vi "Set Properties During Initialization.vi"(6 "Constants VI":path, 8 "error in (no error)":errorcluster, 10 "Properties":T1[](array[typedef]), 11 "Path to VI":path) -> (0 "error out":errorcluster)   [LabVIEW 2017, in "NIVS_Consolidated_CDW_MetaDataObj.lvclass"]
uses:
  NIVS_Consolidated_CDW_MetaDataObj.lvclass
  Property Information.ctl
  <vilib>/Utility/traverseref.llb/TRef TravTarget.ctl
  <vilib>/Utility/traverseref.llb/VI Scripting - Traverse.lvlib
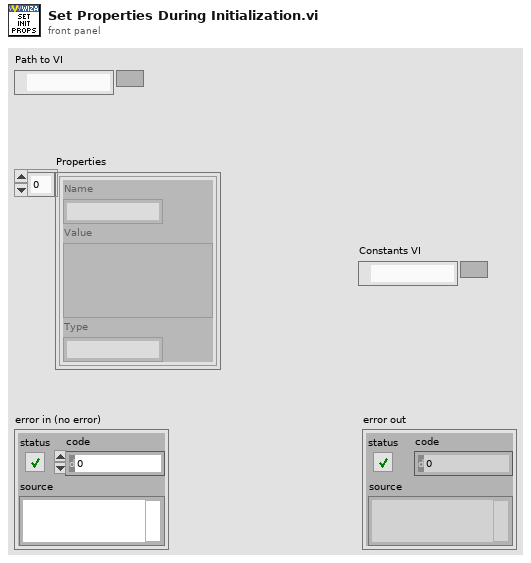
[diagram p1: front panel]
types:
  T1 = typedef "NIVS_Consolidated_CDW_MetaDataObj.lvclass/Property Information.ctl" = cluster{"Name":string, "Value":variant, "Type":string}
  T2 = typedef "TRef TravTarget.ctl" = enum16{"FP", "BD", "Other"}
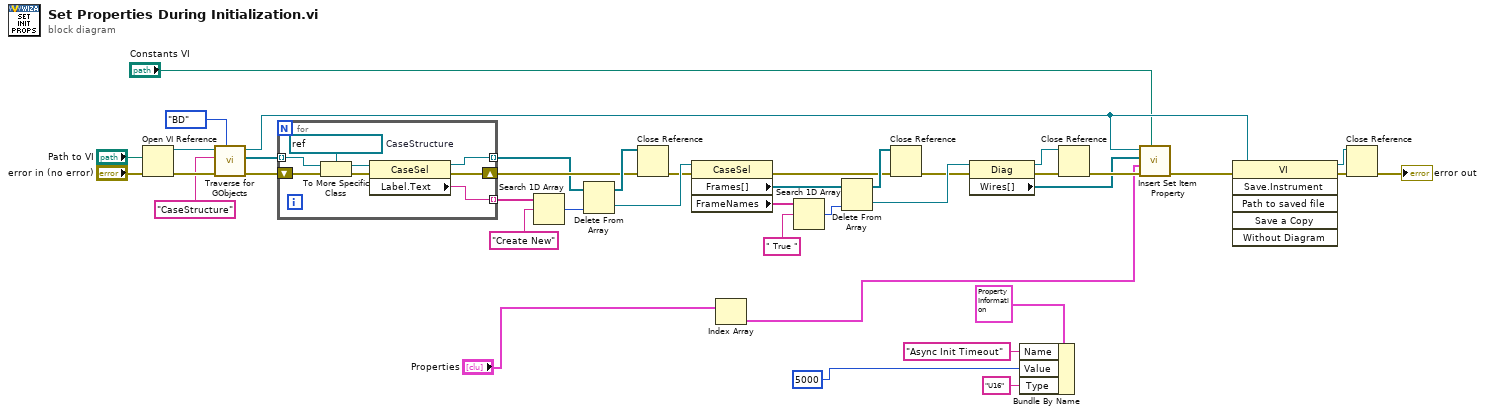
[diagram p0: block diagram]
diagram:
  n1 = Open VI Reference(vi path="Path to VI", error in (no error)="error in (no error)") -> (vi reference=w38:refnum<vi>, error out=w40:errorcluster)  [unwired: 4 in]
  n2 = call <vilib>:"Traverse for GObjects.vi"("Traverse Target"=TRef_TravTarget."BD", "error in (no error)"=w40, "Class Name"="CaseStructure", "VI Refnum"=w38) -> ("error out"=w36:errorcluster, "References"=w33:refnum<vi>[], "dup VI Refnum"=w6:refnum<vi>)  [unwired: 4 in, 1 out]
  n3 = for {
    tunnel: w33 -> [w46] mode=indexing
    shift-right: [w45] -> w30
    shift-left: w36 -> [w47]
    tunnel: [w42] -> w35 mode=indexing
    tunnel: [w41] -> w23 mode=indexing
    w48 = refnum<vi> refnum  # CaseStructure
    n4 = To More Specific Class(target class=w48, reference=w46, error in=w47) -> (specific class reference=w43:refnum<vi>, error out=w44:errorcluster)
    n5 = property class="CaseSel"(reference=w43, error in=w44) -> (reference out=w41:refnum<vi>, error out=w45:errorcluster, "Label.Text"=w42:string)
  }
  n6 = Search 1D Array(1D array=w35, element="Create New") -> (index of element=w31:i32)  [unwired: 1 in]
  n7 = Delete From Array(array=w23, index=w31) -> (deleted portion=w22:refnum<vi>, array with subset deleted=w32:refnum<vi>[])  [unwired: 1 in]
  n8 = Close Reference(reference=w32, error in (no error)=w30) -> (error out=w21:errorcluster)
  n9 = property class="CaseSel"(reference=w22, error in=w21) -> (error out=w20:errorcluster, "Frames[]"=w26:refnum<vi>[], "FrameNames"=w29:string[])  [unwired: 1 out]
  n10 = Index Array(array="Properties") -> (element=w2:T1)  [unwired: 1 in]
  n11 = Search 1D Array(1D array=w29, element=" True ") -> (index of element=w27:i32)  [unwired: 1 in]
  n12 = Delete From Array(array=w26, index=w27) -> (deleted portion=w24:refnum<vi>, array with subset deleted=w25:refnum<vi>[])  [unwired: 1 in]
  n13 = Close Reference(reference=w25, error in (no error)=w20) -> (error out=w19:errorcluster)
  n14 = property class="Diag"(reference=w24, error in=w19) -> (reference out=w15:refnum<vi>, error out=w17:errorcluster, "Wires[]"=w14:refnum<vi>[])
  n15 = Bundle By Name(cluster=T1 {"Name"="", "Value"=variant, "Type"=""} ("Property Info"), "Name"="Async Init Timeout", "Value"=u16 5000, "Type"="U16") -> ()  [unwired: 1 out]
  n16 = Close Reference(reference=w15, error in (no error)=w17) -> (error out=w16:errorcluster)
  n17 = call "Insert Set Item Property.vi"("Constants VI"="Constants VI", "error in (no error)"=w16, "Property Info"=w2, "Wires[]"=w14, "VI Refnum"=w6) -> ("error out"=w4:errorcluster)  [unwired: 5 in, 1 out]
  n18 = invoke class="VI" method="Save.Instrument"(reference=w6, error in=w4) -> (reference out=w5:refnum<vi>, error out=w7:errorcluster)  [unwired: 4 in, 4 out]
  n19 = Close Reference(reference=w5, error in (no error)=w7) -> (error out=→"error out":errorcluster)
